vi "PS Setup.vi"(0 "PS Communication Port":refnum<visa-resource-name>) -> (1 "Units":enum32{"tesla", "kAmps"}(radio) caption="tesla            kAmps", 2 "dup VISA Resource Name":refnum<visa-resource-name>, 3 "Cell":string, 5 "Setpoint":dbl format="%.2f", 6 "Slew Rate":dbl format="%.2f", 7 "error out":errorcluster)   [LabVIEW 2019]
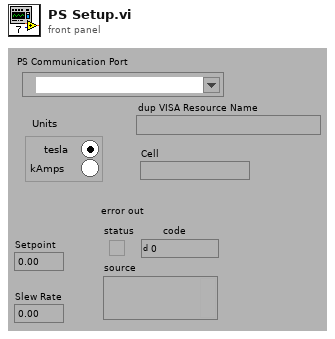
[diagram p1: front panel]
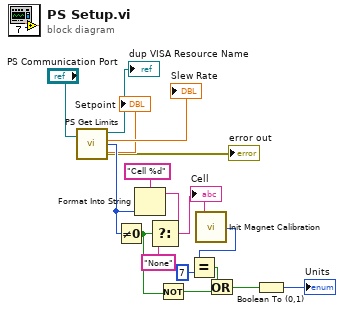
[diagram p0: block diagram]
diagram:
  n1 = call "PS Get Limits.vi"("PS Communication Port"="PS Communication Port") -> ("Setpoint"=→"Setpoint":dbl, "dup VISA Resource Name"=→"dup VISA Resource Name":refnum<visa-resource-name>, "Slew Rate"=→"Slew Rate":dbl, "Cell"=w12:u32, "error out"=→"error out":errorcluster)  [unwired: 2 out]
  n2 = Not Equal To 0?(x=w12) -> (x != 0?=w13:bool)
  n3 = Format Into String(format string="Cell %d", w12) -> (resulting string=w14:string)  [unwired: 2 in, 1 out]
  n4 = Select(t=w14, s=w13, f="None") -> (s? t:f=w16:string)
  "Cell" <- w16
  n5 = Not(x=w13) -> (.not. x?=w17:bool)
  n6 = call "Init Magnet Calibration.vi"("Magnet Id"=w16) -> ("Error Code"=w4:i32)  [unwired: 2 out]
  n7 = Equal?(x=w4, y=7) -> (x = y?=w5:bool)
  n8 = Or(x=w5, y=w17) -> (x .or. y?=w6:bool)
  n9 = Boolean To (0,1)(Boolean=w6) -> (0, 1=→"Units":i16)
